vi "Test HRTF XControl.vi"() -> ()   [LabVIEW 2015]
uses:
  Typedefs/HRTF Config/HRTF Config.xctl
panel:
  out "Mic selection":i32
  in  "stop signal":bool
  in  "flash signal":bool
  in  "complete":i32=-1
  in  "Set file status":bool
  in  "saved":bool[][](array[boolean])
  in  "flash":bool
  in  "highlight":i32=-1
  out "Selection":i32[](array[numeric])
  in  "Get selection":bool
  in  "#speakers":i32
  in  "stop":bool
  in  "HRTF Config":i32(xcontrol)
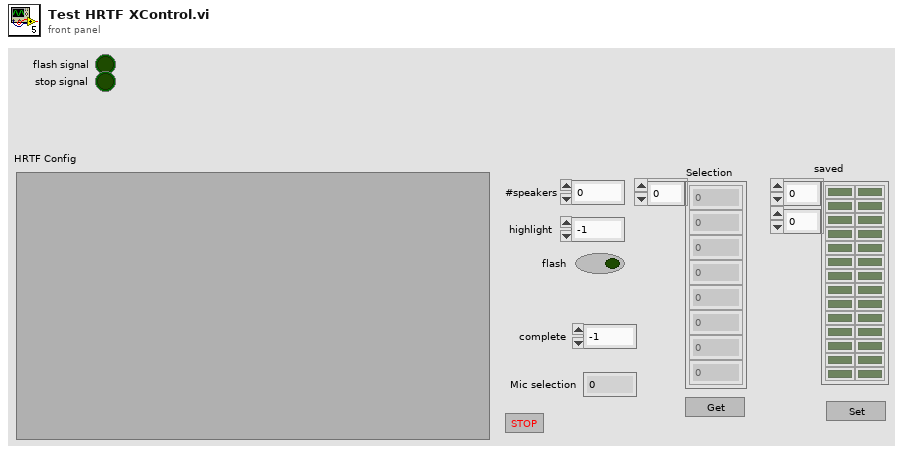
[diagram p1: front panel]
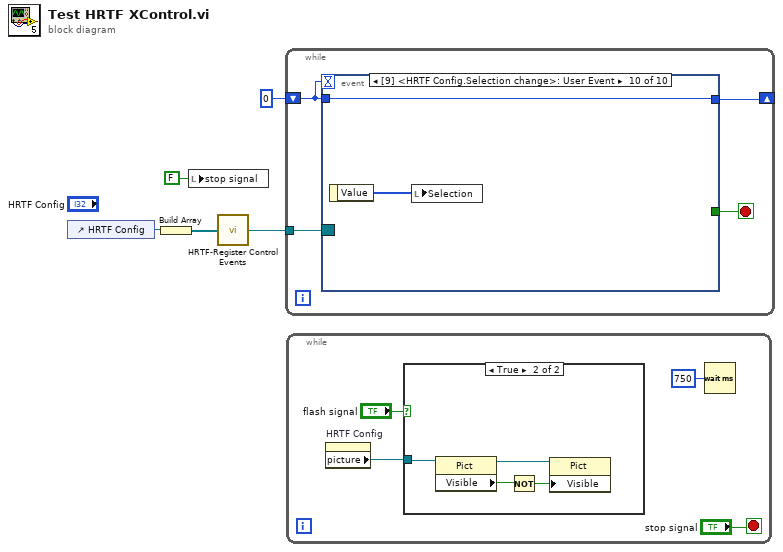
[diagram p0: block diagram]
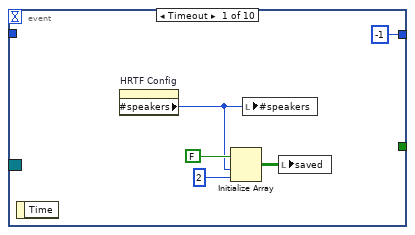
[diagram p3: hidden frame]
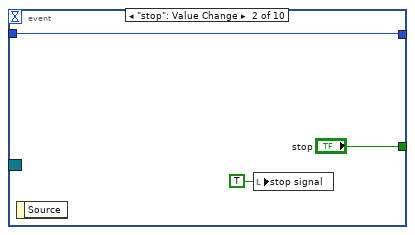
[diagram p4: hidden frame]
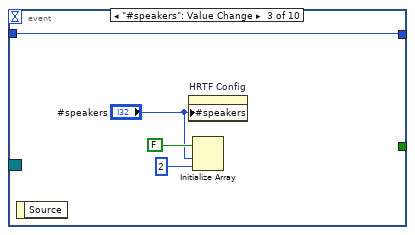
[diagram p5: hidden frame]
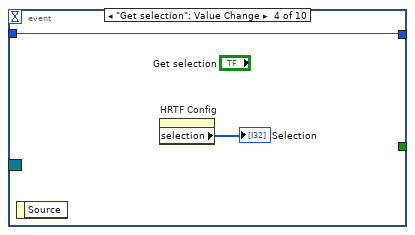
[diagram p6: hidden frame]
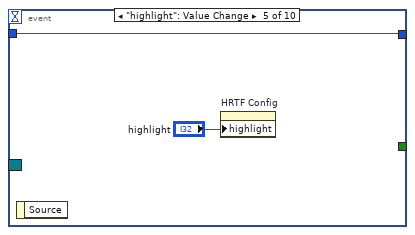
[diagram p7: hidden frame]
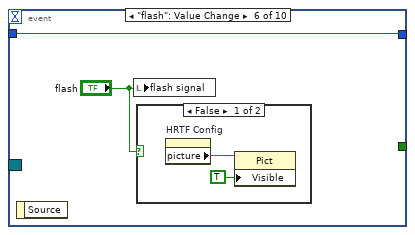
[diagram p8: hidden frame]
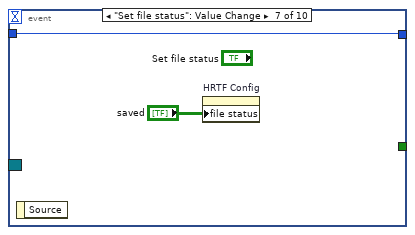
[diagram p10: hidden frame]
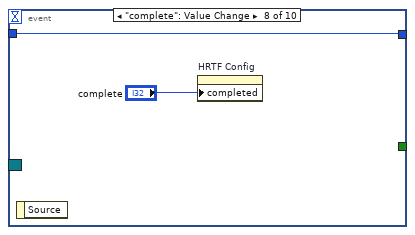
[diagram p11: hidden frame]
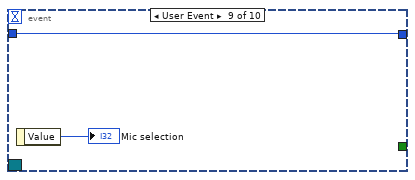
[diagram p12: hidden frame]
diagram:
  n1 = control-ref of="HRTF Config"() -> (w3:refnum<vi>)
  n2 = Build Array(w3) -> (w2:refnum<vi>[])
  n3 = local write "stop signal"(FALSE ("stop signal")) -> ()
  n4 = call "HRTF-Register Control Events.vi"("Refs"=w2) -> ("event registration refnum"=w1:refnum<event-registration>)  [unwired: 13 in, 1 out]
  n5 = while {
    shift-right: [w7] -> _
    shift-left: 0 -> [w8]
    tunnel: w1 -> [w6]
    stop <- w9 stop-if-true
    n6 = event shown="[9] <HRTF Config.Selection change>: User Event" {
      selector: w6 -> [_ _ _ _ _ _ _ _ _ _]
      dyn-events: _ -> [_ _ _ _ _ _ _ _ _ _]
      timeout: w8 -> [_ _ _ _ _ _ _ _ _ _]
      tunnel: [_ "stop" _ _ _ _ _ _ _ _] -> w9
      tunnel: w8 -> [_ w16 w21 w23 w25 w27 w31 w33 w35 w37]
      tunnel: [-1 w16 w21 w23 w25 w27 w31 w33 w35 w37] -> w7
      event Timeout {
        n7 = event-data() -> ()  [unwired: 1 in, 1 out]
        n8 = property on="HRTF Config" class="HRTF Config (strict)"() -> ("#speakers"=w10:i32)  [unwired: 2 in, 2 out]
        n9 = Initialize Array(FALSE, w10, 2 ("dimension size")) -> (w12:bool[][])
        n10 = local write "#speakers"(w10) -> ()
        n11 = local write "saved"(w12) -> ()
      }
      event "stop": Value Change {
        n12 = event-data() -> ()  [unwired: 1 in, 1 out]
        n13 = local write "stop signal"(TRUE ("stop signal")) -> ()
      }
      event "#speakers": Value Change {
        n14 = event-data() -> ()  [unwired: 1 in, 1 out]
        n15 = property on="HRTF Config" class="HRTF Config (strict)"("#speakers"="#speakers") -> ()  [unwired: 2 in, 2 out]
        n16 = Initialize Array(FALSE, "#speakers", 2 ("dimension size")) -> ()  [unwired: 1 out]
      }
      event "Get selection": Value Change {
        n17 = event-data() -> ()  [unwired: 1 in, 1 out]
        n18 = property on="HRTF Config" class="HRTF Config (strict)"() -> ("selection"=→"Selection":i32[])  [unwired: 2 in, 2 out]
      }
      event "highlight": Value Change {
        n19 = event-data() -> ()  [unwired: 1 in, 1 out]
        n20 = property on="HRTF Config" class="HRTF Config (strict)"("highlight"="highlight") -> ()  [unwired: 2 in, 2 out]
      }
      event "flash": Value Change {
        n21 = event-data() -> ()  [unwired: 1 in, 1 out]
        n22 = local write "flash signal"("flash") -> ()
        n23 = case shown="False" "flash" {
          frame False {
            n24 = property on="HRTF Config" class="HRTF Config (strict)"() -> ("picture"=w29:refnum<vi>)  [unwired: 2 in, 2 out]
            n25 = property class="Pict"(reference=w29, "Visible"=TRUE) -> ()  [unwired: 1 in, 2 out]
          }
          frame True {
          }
        }
      }
      event "Set file status": Value Change {
        n26 = event-data() -> ()  [unwired: 1 in, 1 out]
        n27 = property on="HRTF Config" class="HRTF Config (strict)"("file status"="saved") -> ()  [unwired: 2 in, 2 out]
      }
      event "complete": Value Change {
        n28 = event-data() -> ()  [unwired: 1 in, 1 out]
        n29 = property on="HRTF Config" class="HRTF Config (strict)"("completed"="complete") -> ()  [unwired: 2 in, 2 out]
      }
      event User Event {
        n30 = event-data() -> ("Value"=→"Mic selection":i32)  [unwired: 1 in]
      }
      event User Event {
        n31 = event-data() -> ("Value"=w36:i32[])  [unwired: 1 in]
        n32 = local write "Selection"(w36) -> ()
      }
    }
  }
  n33 = while {
    stop <- "stop signal" stop-if-true
    n34 = property on="HRTF Config" class="HRTF Config (strict)"() -> ("picture"=w40:refnum<vi>)  [unwired: 2 in, 2 out]
    n35 = case shown="True" "flash signal" {
      tunnel: w40 -> [_ w45]
      frame False {
      }
      frame True {
        n36 = property class="Pict"(reference=w45) -> (reference out=w44:refnum<vi>, "Visible"=w43:bool)  [unwired: 1 in, 1 out]
        n37 = Not(x=w43) -> (.not. x?=w42:bool)
        n38 = property class="Pict"(reference=w44, "Visible"=w42) -> ()  [unwired: 1 in, 2 out]
      }
    }
    n39 = Wait (ms)(milliseconds to wait=u32 750) -> ()  [unwired: 1 out]
  }
